vi "Interface_Asset_Write Process Name.vi"(10 "Process Name":string, 11 "Grid in":refnum<class "Grid.lvclass">) -> (3 "Grid out":refnum<class "Grid.lvclass">)   [LabVIEW 2015, in "Grid.lvclass"]
uses:
  Grid.lvclass
  Grid.lvclass/Grid.ctl
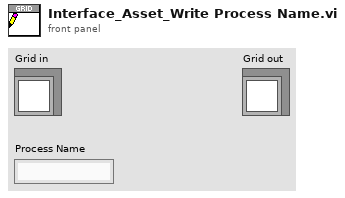
[diagram p1: front panel]
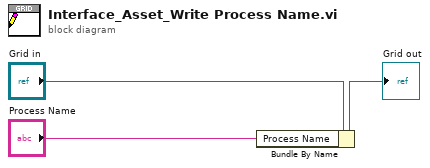
[diagram p0: block diagram]
diagram:
  n1 = Bundle By Name(cluster="Grid in", "Process Name"="Process Name") -> (→"Grid out":refnum<class "Grid.lvclass">)
